vi "Statistics.vi"() -> ()   [LabVIEW 2011]
doc: "This example shows the results of statistical functions. There is a Histogram of all values and there is the Minimum, Maximum and Mean for each packet of data.\n\nThis example uses the following Express VIs: Simulate Signal, Create Histogram, and Statistics."
uses:
  Instance           4 18Saved   Statistics .vi
  Instance           1 18Saved   Statistics .vi
  Instance           3 18Saved   Statistics .vi
  Instance           2 18Saved   Statistics .vi
panel:
  out "Chart":dynamicdata(graph)
  out "Mean":dbl format="%0.4f"
  out "Minimum":dbl format="%0.4f"
  out "Maximum":dbl format="%0.4f"
  out "Signal":dynamicdata(graph)
  out "Histogram":dynamicdata(graph)
  in  "stop":bool
  # "This example shows the results of statistical functions.\nThere is a Histogram of all values and there is the Minimum, Maximum and Mean for each packet of data."
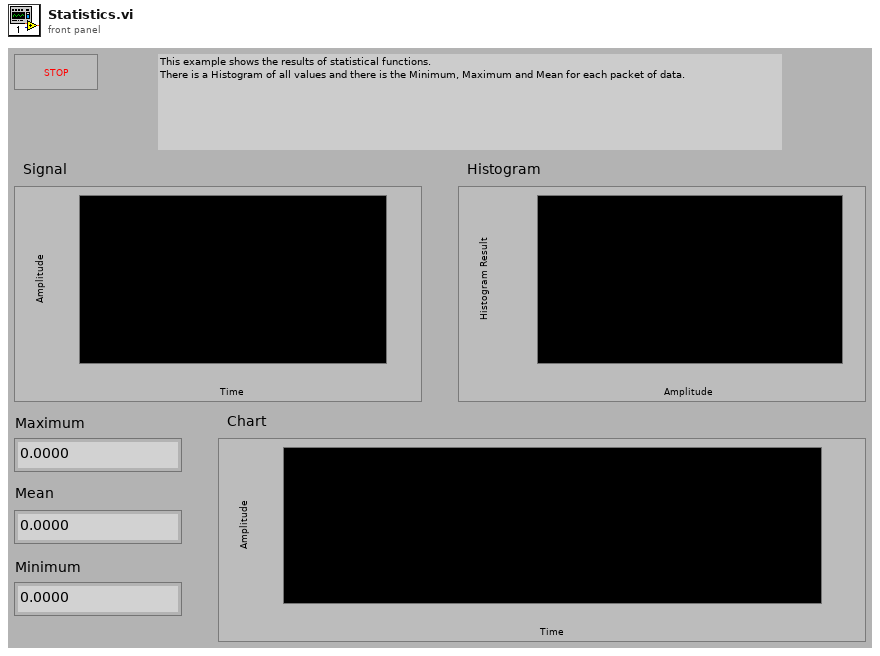
[diagram p1: front panel]
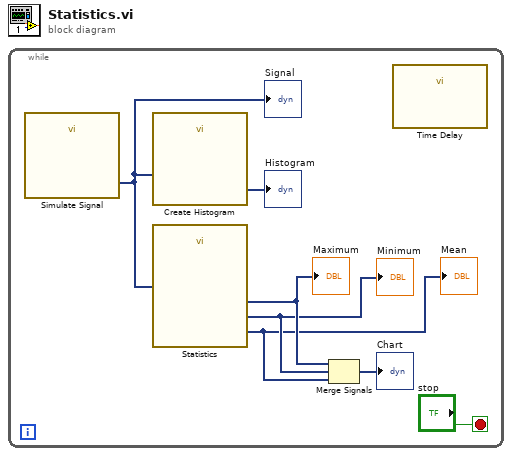
[diagram p0: block diagram]
diagram:
  n1 = while {
    stop <- "stop" stop-if-true
    n2 = call "Simulate Signal"() -> ("DC with Gaussian Noise"=w4:dynamicdata)  [unwired: 14 in, 1 out]
    "Signal" <- w4
    n3 = call "Create Histogram"("Signal"=w4) -> ("Histogram"=→"Histogram":dynamicdata)  [unwired: 9 in, 1 out]
    n4 = call "Statistics"("Signals"=w4) -> ("Arithmetic Mean"=w1:dynamicdata, "Minimum"=w2:dynamicdata, "Maximum"=w3:dynamicdata)  [unwired: 23 in, 1 out]
    "Maximum" <- w3
    "Minimum" <- w2
    "Mean" <- w1
    n5 = Merge Signals(w3, w2, w1) -> (→"Chart":dynamicdata)
    n6 = call "Time Delay"() -> ()  [unwired: 11 in, 1 out]
  }
